vi "ComputeShifts.vi"(0 "Scan Plane Data":dbl[][][](array[numeric]), 1 "FFT size":i32=256, 2 "Ref Horizontal SF Phase":dbl, 3 "Ref Row Shift Element":dbl, 4 "Ref Vertical SF Phase":dbl, 5 "Ref Col Shift Element":dbl, 7 "Header":T1) -> (14 "Row Shift Array":dbl[](array[numeric]), 17 "Col Shift Array":dbl[](array[numeric]))   [LabVIEW 2014]
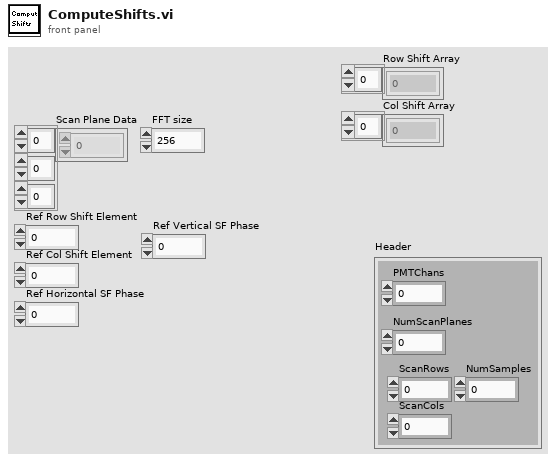
[diagram p1: front panel]
types:
  T1 = cluster{"PMTChans":i32, "NumScanPlanes":i32, "ScanRows":i32, "ScanCols":i32, "NumSamples":i32}
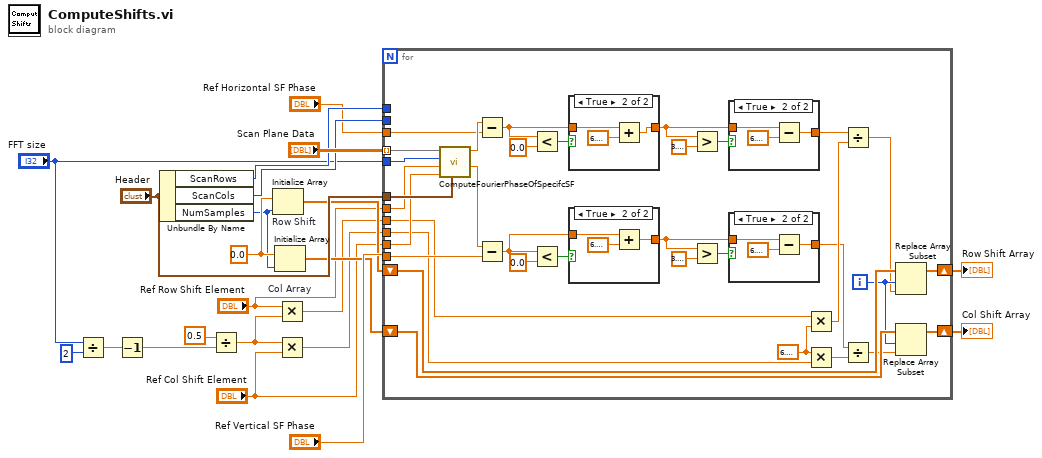
[diagram p0: block diagram]
diagram:
  w19 = 0.0 ("element")
  n1 = Divide(x="FFT size", y=2) -> (x/y=w10:dbl)
  n2 = Decrement(x=w10) -> (x-1=w9:dbl)
  n3 = Unbundle By Name("Header") -> ("ScanRows"=w21:i32, "ScanCols"=w20:i32, "NumSamples"=w18:i32)
  n4 = Divide(x=0.5, y=w9) -> (x/y=w6:dbl)
  n5 = Initialize Array "Row Shift"(w19, w18) -> (w14:dbl[])
  n6 = Initialize Array "Col Array"(w19, w18) -> (w13:dbl[])
  n7 = Multiply(x="Ref Row Shift Element", y=w6) -> (x*y=w4:dbl)
  n8 = Multiply(x=w6, y="Ref Col Shift Element") -> (x*y=w3:dbl)
  n9 = for {
    tunnel: "Scan Plane Data" -> [w57] mode=indexing
    tunnel: w21 -> [_]
    tunnel: w20 -> [_]
    tunnel: "Header" -> [w55]
    tunnel: "FFT size" -> [w56]
    tunnel: "Ref Row Shift Element" -> [w54]
    tunnel: "Ref Col Shift Element" -> [w53]
    tunnel: "Ref Horizontal SF Phase" -> [w50]
    tunnel: "Ref Vertical SF Phase" -> [w49]
    shift-right: [w35] -> w2
    shift-left: w14 -> [w36]
    shift-right: [w33] -> w1
    shift-left: w13 -> [w34]
    tunnel: w4 -> [w31]
    tunnel: w3 -> [w29]
    i -> [w32]
    w30 = 6.283185307179586
    n10 = call "ComputeFourierPhaseOfSpecifcSF.vi"("Header"=w55, "Col Element Number"=w53, "Row Element Numbert"=w54, "FFT size"=w56, "Scan Frame"=w57) -> ("Vertical SF Phase"=w51:dbl, "Horizontal SF Phase"=w52:dbl)  [unwired: 3 in]
    n11 = Subtract(x=w52, y=w50) -> (x-y=w45:dbl)
    n12 = Subtract(x=w51, y=w49) -> (x-y=w43:dbl)
    n13 = Less?(x=w45, y=0.0) -> (x < y?=w46:bool)
    n14 = Less?(x=w43, y=0.0) -> (x < y?=w44:bool)
    n15 = case shown="True" w46 {
      tunnel: w45 -> [w70 w72]
      tunnel: [w70 w71] -> w40
      frame False {
      }
      frame True {
        n16 = Add(x=w72, y=6.283185307179586) -> (x+y=w71:dbl)
      }
    }
    n17 = case shown="True" w44 {
      tunnel: w43 -> [w66 w68]
      tunnel: [w66 w67] -> w37
      frame False {
      }
      frame True {
        n18 = Add(x=w68, y=6.283185307179586) -> (x+y=w67:dbl)
      }
    }
    n19 = Greater?(x=w40, y=3.141592653589793) -> (0:w41:bool)
    n20 = Greater?(x=w37, y=3.141592653589793) -> (0:w38:bool)
    n21 = case shown="True" w41 {
      tunnel: w40 -> [w62 w64]
      tunnel: [w62 w63] -> w27
      frame False {
      }
      frame True {
        n22 = Subtract(x=w64, y=6.283185307179586) -> (x-y=w63:dbl)
      }
    }
    n23 = case shown="True" w38 {
      tunnel: w37 -> [w58 w60]
      tunnel: [w58 w59] -> w25
      frame False {
      }
      frame True {
        n24 = Subtract(x=w60, y=6.283185307179586) -> (x-y=w59:dbl)
      }
    }
    n25 = Multiply(x=w31, y=w30) -> (x*y=w28:dbl)
    n26 = Multiply(x=w30, y=w29) -> (x*y=w26:dbl)
    n27 = Divide(x=w27, y=w28) -> (x/y=w24:dbl)
    n28 = Divide(x=w25, y=w26) -> (x/y=w23:dbl)
    n29 = Replace Array Subset(array=w36, new element=w24, index=w32) -> (w35:dbl[])
    n30 = Replace Array Subset(array=w34, new element=w23, index=w32) -> (w33:dbl[])
  }
  "Row Shift Array" <- w2
  "Col Shift Array" <- w1
